vi "data send (SubVI).vi"(11 "보내기":T1={"국번"="0", "커맨드"="01", "데이터 No."="00", "데이터"="00"}) -> (3 "문자열":string)   [LabVIEW 2014]
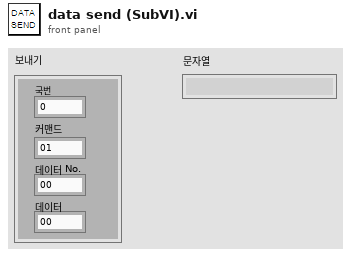
[diagram p1: front panel]
types:
  T1 = cluster{"국번":string, "커맨드":string, "데이터 No.":string, "데이터":string}
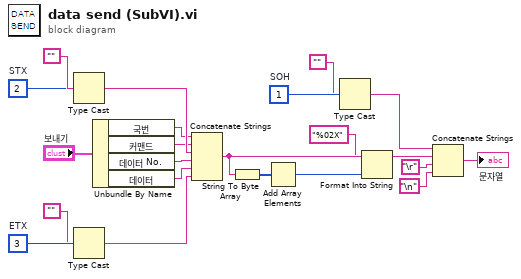
[diagram p0: block diagram]
diagram:
  w16 = u8 3  # ETX
  w12 = u8 2  # STX
  w7 = u8 1  # SOH
  n1 = Type Cast(type="", x=w12) -> (*(type *) &x=w14:string)
  n2 = Type Cast(type="", x=w16) -> (*(type *) &x=w17:string)
  n3 = Unbundle By Name("보내기") -> ("국번"=w4:string, "커맨드"=w3:string, "데이터 No."=w2:string, "데이터"=w1:string)
  n4 = Concatenate Strings(w4, w3, w14, w2, w1, w17) -> (w11:string)
  n5 = String To Byte Array(string=w11) -> (unsigned byte array=w8:u8[])
  n6 = Add Array Elements(numeric array=w8) -> (sum=w9:u8)
  n7 = Type Cast(type="", x=w7) -> (*(type *) &x=w18:string)
  n8 = Format Into String(format string="%02X", initial string=w11, w9) -> (resulting string=w19:string)  [unwired: 1 in, 1 out]
  n9 = Concatenate Strings(w18, w19, "\r", "\n") -> (→"문자열":string)
